vi "http parse header.vi"(9 "handler queue":refnum<queue>, 10 "data in":string, 11 "application request":T1) -> (2 "abort":bool, 3 "application request out":T1)   [LabVIEW 2016, in "Basic HTTP server.lvclass"]
uses:
  Basic HTTP server.lvclass
  http request.ctl
  http method.ctl
  HTTP headers/http header data.ctl
  <vilib>/dlg_ctls.llb/Space Constant.vi
  HTTP headers/http add header to set.vi
  HTTP headers/http headers.lvlib
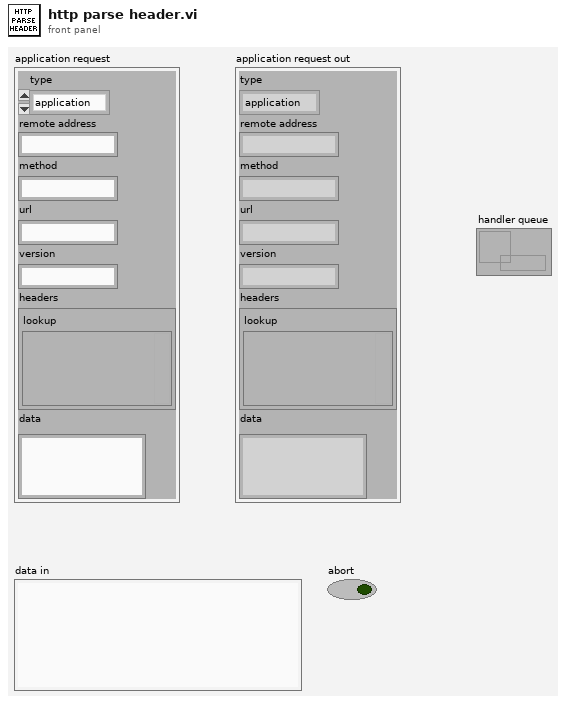
[diagram p1: front panel]
types:
  T1 = typedef "Basic HTTP server.lvclass/http request.ctl" = cluster{"type":T2, "remote address":string, "method":string, "url":string, "version":string, "headers":T3, "data":string}
  T2 = typedef "Basic HTTP server.lvclass/http method.ctl" = enum16{"application", "error", "upgrade", "expect"}
  T3 = typedef "http headers.lvlib/http header data.ctl" = cluster{"lookup":variant}
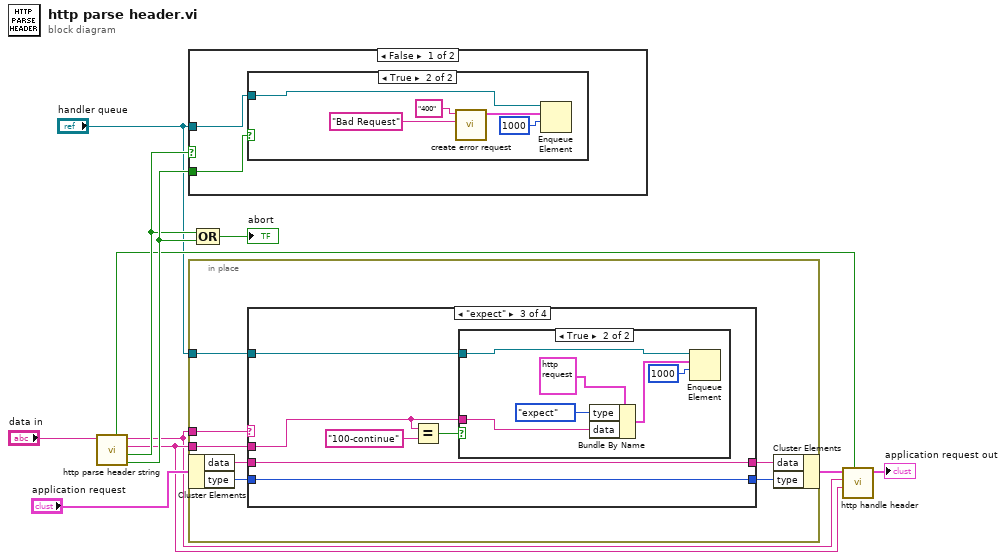
[diagram p0: block diagram]
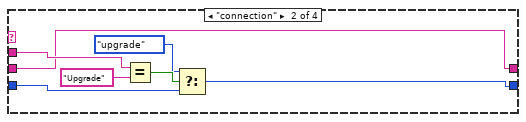
[diagram p3: hidden frame]
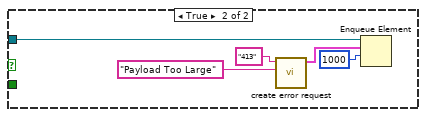
[diagram p7: hidden frame]
diagram:
  n1 = call "http parse header string.vi"("raw string"="data in") -> ("no field name"=w8:bool, "no crlf"=w7:bool, "header field data"=w4:string, "header field name"=w3:string, "continuation"=w2:bool)  [unwired: 6 in]
  n2 = case shown="False" w7 {
    tunnel: w8 -> [w13 _]
    tunnel: "handler queue" -> [w12 w23]
    frame False {
      n3 = case shown="True" w13 {
        tunnel: w12 -> [_ w14]
        frame False {
        }
        frame True {
          n4 = call "create error request.vi"("reason"="Bad Request" ("status string"), "code"="400") -> ("element"=w18:T1)  [unwired: 9 in]
          n5 = Enqueue Element(queue=w14, element=w18, timeout in ms (-1)=1000) -> ()  [unwired: 1 in, 3 out]
        }
      }
    }
    frame True {
      n6 = call "create error request.vi"("reason"="Payload Too Large" ("status string"), "code"="413") -> ("element"=w22:T1)  [unwired: 9 in]
      n7 = Enqueue Element(queue=w23, element=w22, timeout in ms (-1)=1000) -> ()  [unwired: 1 in, 3 out]
    }
  }
  n8 = in-place {
    in-place-border: w3 -> [w30]
    in-place-border: w4 -> [w27]
    in-place-border: "handler queue" -> [w24]
    n9 = in-place-cluster #1("application request") -> ("data"=w28:string, "type"=w25:T2)
    n10 = case shown="\"expect\"" w30 {
      selector: w30 -> [w32 _ _ _]
      tunnel: [w32 w33 w45 w53] -> w29
      tunnel: w28 -> [_ w33 w45 w53]
      tunnel: w27 -> [_ w38 w40 _]
      tunnel: [w31 w35 w44 w52] -> w26
      tunnel: w25 -> [w31 w34 w44 w52]
      tunnel: w24 -> [_ _ w41 _]
      frame "content-length", "transfer-encoding" {
      }
      frame "connection" {
        n11 = Equal?(x=w38, y="Upgrade" ("name")) -> (x = y?=w37:bool)
        n12 = Select(t=http_method."upgrade", s=w37, f=w34) -> (s? t:f=w35:T2)
      }
      frame "expect" {
        n13 = Equal?(x=w40, y="100-continue") -> (x = y?=w42:bool)
        n14 = case shown="True" w42 {
          tunnel: w41 -> [_ w51]
          tunnel: w40 -> [_ w46]
          frame False {
          }
          frame True {
            n15 = Bundle By Name(cluster=T1 {"type"=enum."application", "remote address"="", "method"="", "url"="", "version"="", "headers"={"lookup"=variant}, "data"=""} ("element"), "type"=http_method."expect", "data"=w46) -> (w49:T1)
            n16 = Enqueue Element(queue=w51, element=w49, timeout in ms (-1)=1000) -> ()  [unwired: 1 in, 3 out]
          }
        }
      }
      frame Default {
      }
    }
    n17 = in-place-cluster #1("data"=w29, "type"=w26) -> (w6:T1)
  }
  n18 = Compound Arithmetic op=OR(w7, w8) -> (→"abort":bool)
  n19 = call "http handle header.vi"("continuation"=w2, "header field data"=w4, "header field name"=w3, "application request in"=w6) -> ("application request out"=→"application request out":T1)  [unwired: 7 in]
